vi "ENED 1100 Task 2A CFU 9 29.vi"() -> ()   [LabVIEW 2016]
panel:
  out "End Value":dbl
  in  "End":dbl
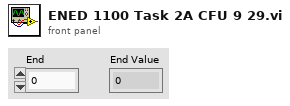
[diagram p1: front panel]
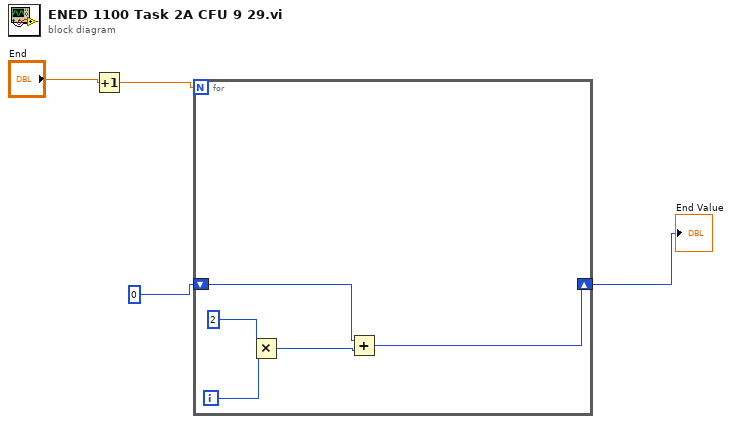
[diagram p0: block diagram]
diagram:
  n1 = Increment(x="End") -> (x+1=w3:dbl)
  n2 = for {
    N: w3 -> [_]
    shift-right: [w5] -> w1
    shift-left: 0 -> [w7]
    i -> [w8]
    n3 = Multiply(x=2, y=w8) -> (x*y=w6:i32)
    n4 = Add(x=w7, y=w6) -> (x+y=w5:i32)
  }
  "End Value" <- w1
